vi "System Check.vi"(8 "Error In":errorcluster) -> (0 "Error Out":errorcluster)   [LabVIEW 2019, in "LMH-LINX.lvlib"]
uses:
  <vilib>/MakerHub/LINX/LMH-LINX.lvlib
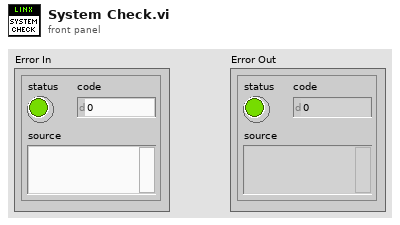
[diagram p1: front panel]
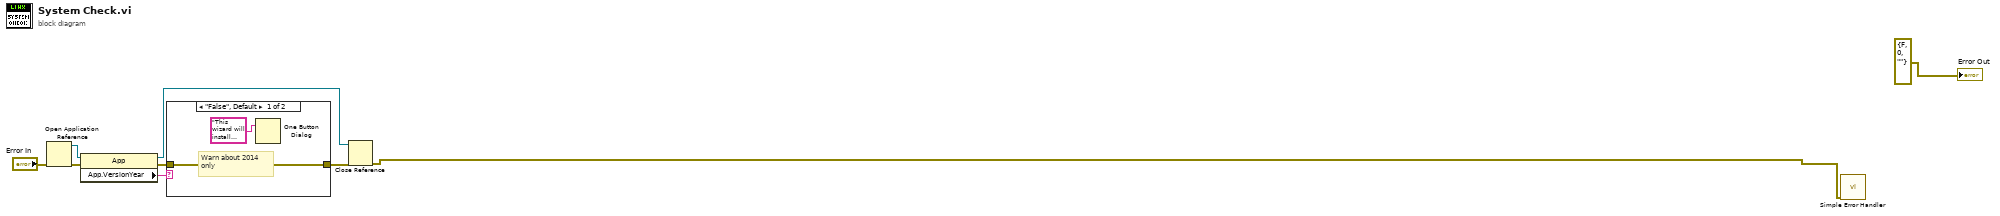
[diagram p0: block diagram]
diagram:
  n1 = Open Application Reference(8:"Error In") -> (0:w6:errorcluster, 3:w8:refnum<vi>)  [unwired: 3 in]
  n2 = property class="App"(reference=w8, error in=w6) -> (reference out=w7:refnum<vi>, error out=w3:errorcluster, "App.VersionYear"=w5:string)
  n3 = case shown="\"False\", Default" w5 {
    tunnel: [w11 w12] -> w4
    tunnel: w3 -> [w11 w12]
    frame "False", Default {
      # "Warn about 2014\nonly"
      n4 = One Button Dialog(message="This wizard will install LabVIEW 2014 support to the target device.  \nYou will only be able to connect to and use the device from LabVIEW 2014.") -> ()  [unwired: 1 in, 1 out]
    }
    frame "2014" {
    }
  }
  n5 = Close Reference(reference=w7, error in (no error)=w4) -> (error out=w2:errorcluster)
  n6 = call <vilib>:"Simple Error Handler.vi"("error in (no error)"=w2) -> ()  [unwired: 4 in, 5 out]
  "Error Out" <- errorcluster {"status"=FALSE, "code"=0, "source"=""} ("error constant")
